vi "FPTempEx.vi"() -> ()   [LabVIEW 2010]
uses:
  Instance           1 16Saved   FPTempEx .vi
  Instance           2 16Saved   FPTempEx .vi
panel:
  out "Array":dbl[](array[numeric])
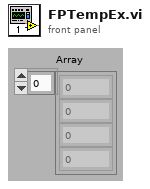
[diagram p1: front panel]
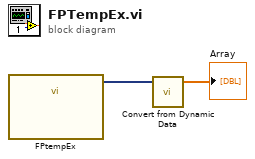
[diagram p0: block diagram]
diagram:
  n1 = call "FPtempEx"() -> ("Value out"=w2:dynamicdata)  [unwired: 5 in, 2 out]
  n2 = call "Convert from Dynamic Data"("Dynamic Data Type"=w2) -> ("Array"=→"Array":dbl[])  [unwired: 3 in]
